vi "Calculate Off Channel Amplitude.vi"(11 "Waveform Array":waveform(dbl)[](array[waveform])) -> (0 "error out":errorcluster, 3 "Pulse Amplitudes":dbl[](array[numeric]))   [LabVIEW 2010]
uses:
  <vilib>/measure/mamon.llb/Trigger Detection for 1 Channel.vi
  <vilib>/Analysis/NI_AALBase.lvlib
  <vilib>/measure/NI_MAPro.lvlib
panel:
  out "Waveform Array 2":waveform(dbl)[](graph)
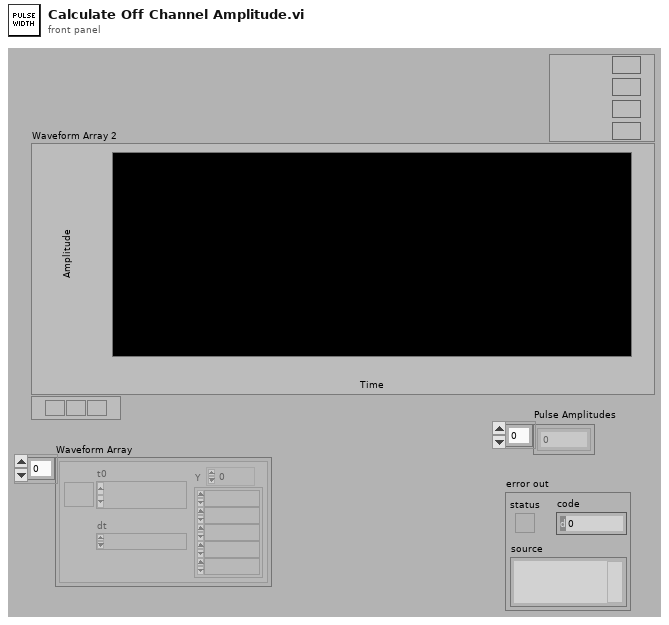
[diagram p1: front panel]
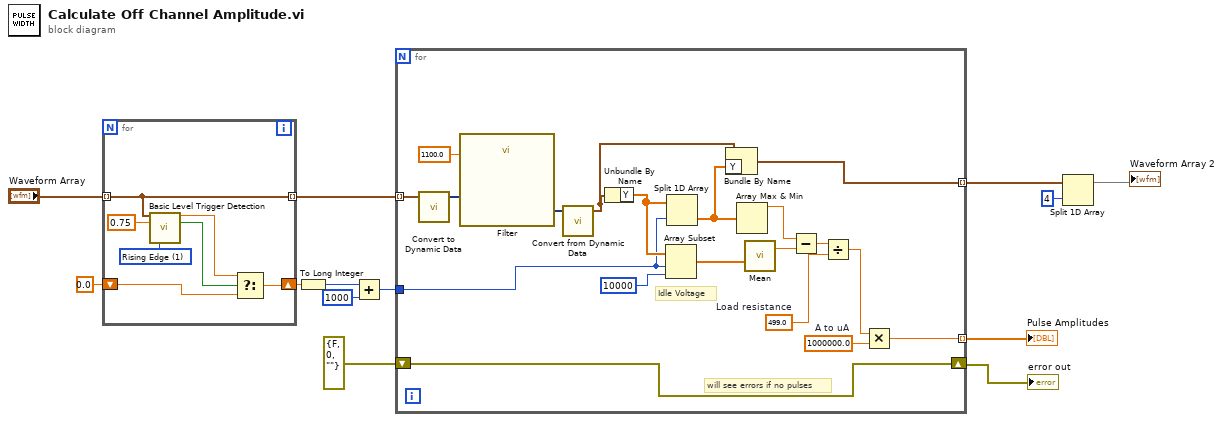
[diagram p0: block diagram]
diagram:
  n1 = for {
    tunnel: "Waveform Array" -> [w20] mode=indexing
    tunnel: [w20] -> w6 mode=indexing
    shift-right: [w17] -> w3
    shift-left: 0.0 ("trigger location") -> [w14]
    w18 = u16 1 items=["Falling Edge", "Rising Edge"] ("trigger slope")
    n2 = call-poly <vilib>:"Basic Level Trigger Detection.vi"("signal in"=w20, "level"=0.75, "trigger slope"=w18) -> ("trigger location"=w15:dbl, "trigger detected?"=w16:bool)  [unwired: 10 in, 1 out]
    n3 = Select(t=w15, s=w16, f=w14) -> (s? t:f=w17:dbl)
  }
  n4 = To Long Integer(number=w3) -> (32bit integer=w2:i32)
  n5 = Add(x=w2, y=1000 ("index")) -> (x+y=w1:i32)
  n6 = for {
    tunnel: w6 -> [w27] mode=indexing
    tunnel: [w34] -> w11 mode=indexing
    shift-right: [w39] -> w13
    shift-left: errorcluster {"status"=FALSE, "code"=0, "source"=""} ("error out") -> [w39]
    tunnel: [w21] -> w8 mode=indexing
    tunnel: w1 -> [w24]
    w33 = 1000000.0  # A to uA
    w36 = 499.0  # Load resistance
    # "Idle Voltage"
    # "will see errors if no pulses"
    n7 = call "Convert to Dynamic Data"("Waveform"=w27) -> ("Dynamic Data Type"=w28:dynamicdata)  [unwired: 3 in]
    n8 = call "Filter"("Lower Cut-Off"=1100.0, "Signal"=w28) -> ("Filtered Signal"=w29:dynamicdata)  [unwired: 8 in, 1 out]
    n9 = call "Convert from Dynamic Data"("Dynamic Data Type"=w29) -> ("Waveform"=w23:waveform(dbl))  [unwired: 3 in]
    n10 = Unbundle By Name(w23) -> ("Y"=w32:dbl[])
    n11 = Array Subset(array=w32, index=w24, length=10000) -> (w31:dbl[])
    n12 = Split 1D Array(array=w32, index=w24) -> (second subarray=w22:dbl[])  [unwired: 1 out]
    n13 = Bundle By Name(cluster=w23, "Y"=w22) -> (w21:waveform(dbl))
    n14 = Array Max & Min(array=w22) -> (max value=w38:dbl)  [unwired: 3 out]
    n15 = call <vilib>:"Mean.vi"("X"=w31) -> ("mean"=w30:dbl)  [unwired: 1 out]
    n16 = Subtract(x=w38, y=w30) -> (x-y=w37:dbl)
    n17 = Divide(x=w37, y=w36) -> (x/y=w35:dbl)
    n18 = Multiply(x=w35, y=w33) -> (x*y=w34:dbl)
  }
  "error out" <- w13
  "Pulse Amplitudes" <- w11
  n19 = Split 1D Array(array=w8, index=4) -> (first subarray=→"Waveform Array 2":waveform(dbl)[])  [unwired: 1 out]
